vi "FGV_Reference.vi"(7 "FV_Acquire":enum16{"Set", "Get"}(ring), 9 "Real Rate In":dbl, 10 "CoilVolte In":refnum<k21>, 11 "LineEncoder  In":refnum<k21>) -> (1 "Real Rate Out":dbl, 2 "CoilVolte Out":refnum<k21>, 3 "LineEncoder Out":refnum<k21>)   [LabVIEW 2017]
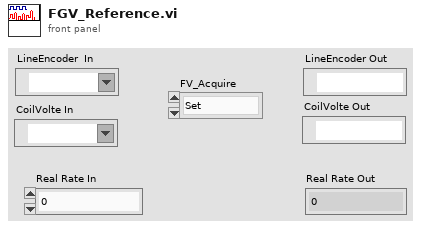
[diagram p1: front panel]
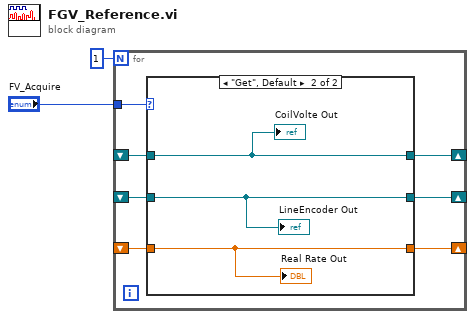
[diagram p0: block diagram]
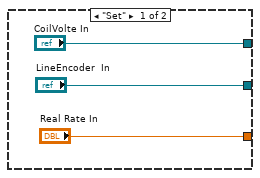
[diagram p2: hidden frame]
diagram:
  n1 = for {
    N: 1 -> [_]
    tunnel: "FV_Acquire" -> [w9]
    shift-right: [w8] -> _
    shift-left: _ -> [w6]
    shift-right: [w7] -> _
    shift-left: _ -> [w5]
    shift-right: [w4] -> _
    shift-left: _ -> [w3]
    n2 = case shown="\"Get\", Default" w9 {
      tunnel: ["CoilVolte In" w15] -> w8
      tunnel: ["LineEncoder  In" w14] -> w7
      tunnel: w6 -> [_ w15]
      tunnel: w5 -> [_ w14]
      tunnel: ["Real Rate In" w13] -> w4
      tunnel: w3 -> [_ w13]
      frame "Set" {
      }
      frame "Get", Default {
        "CoilVolte Out" <- w15
        "LineEncoder Out" <- w14
        "Real Rate Out" <- w13
      }
    }
  }
